vi "mprintf.vi"(8 "error in (no error)":errorcluster, 10 "para1":u64, 11 "para0":string) -> (0 "error out":errorcluster, 3 "function return":string)   [LabVIEW 2020, in "sqlite3.lvlib"]
uses:
  sqlite3.lvlib
  errstr.vi
  bin/sqlite3_64.dll
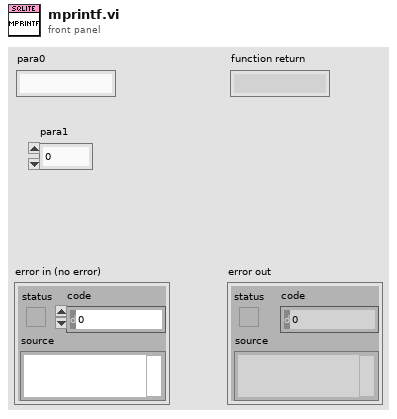
[diagram p1: front panel]
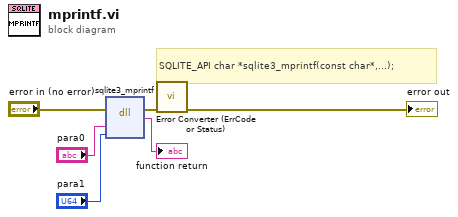
[diagram p0: block diagram]
diagram:
  # "SQLITE_API char *sqlite3_mprintf(const char*,...);"
  n1 = dll-call lib="C:/Users/Fred.Guo/Desktop/Database-configuration/externals/sqlite3/Source/bin/sqlite3_*.*" fn="sqlite3_mprintf"(error in="error in (no error)", "para0"="para0", "para1"="para1") -> (error out=w2:errorcluster, →"function return":string)  [unwired: 4 in, 1 out]
  n2 = call "Error Converter (ErrCode or Status).vi"("error in (no error)"=w2) -> ("error out"=→"error out":errorcluster)  [unwired: 10 in]
